vi "Test Virtual Thermometer from CSV.vi"(11 "Test Case In":refnum<class "Test Instrument Manager.lvclass">) -> (0 "error out":errorcluster, 3 "Test Case Out":refnum<class "Test Instrument Manager.lvclass">)   [LabVIEW 2024, in "Test Instrument Manager.lvclass"]
uses:
  Test Instrument Manager.lvclass
  Test Instrument Manager.lvclass/Test Instrument Manager.ctl
  Source/Instrument Manager/Instrument Manager.lvclass
  Source/Interfaces/IRead Temperature/IRead Temperature.lvclass
  Source/Interfaces/IVirtual Instrument/IVirtual Instrument.lvclass
  <vilib>/Astemes/LUnit/Test Case.lvclass
  cceb4bd8-3600-4d38-a702-34d5b4246d90.vi
panel:
  out "Time Stamp":timestamp format="%<%x %.3X>T"
  out "Waveform Chart":dbl(graph)
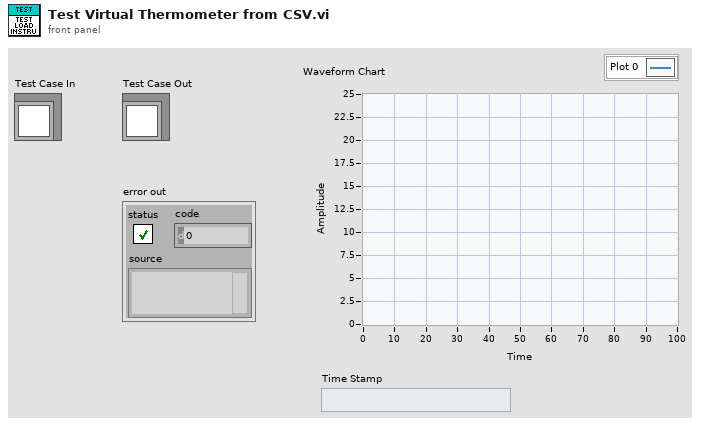
[diagram p1: front panel]
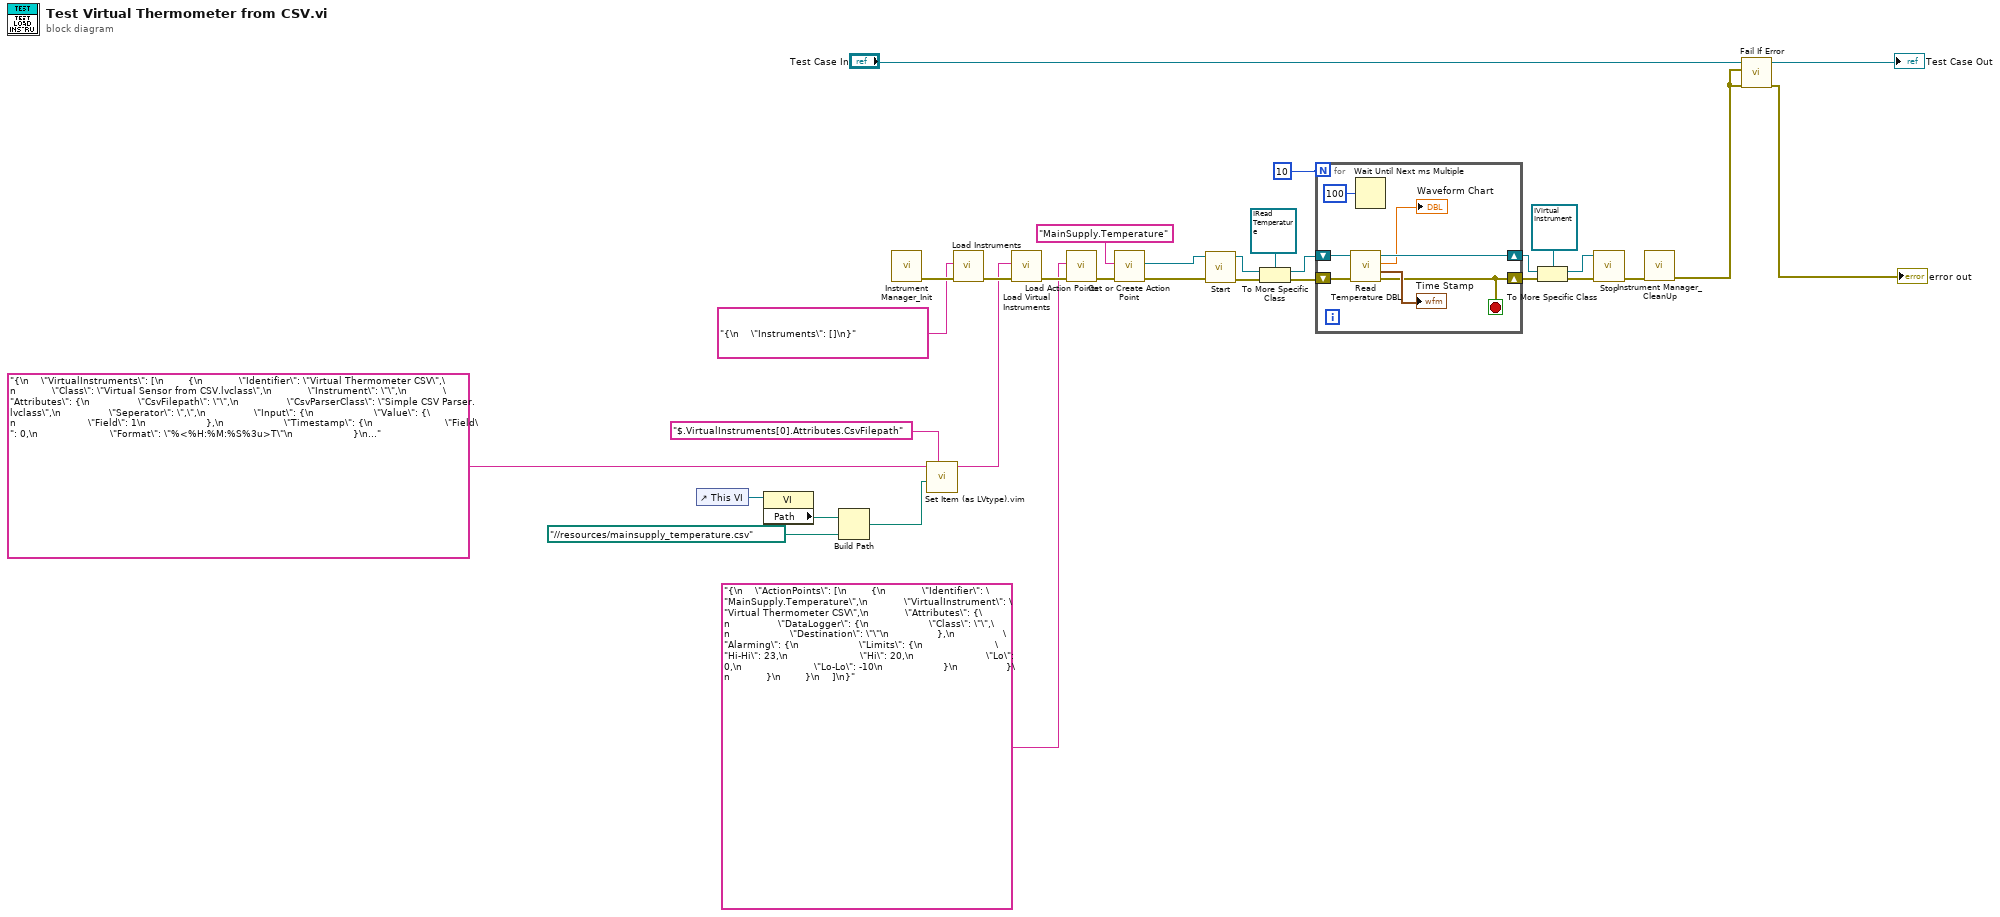
[diagram p0: block diagram]
diagram:
  n1 = control-ref of="This VI"() -> (w5:refnum<vi>)
  n2 = property class="VI"(reference=w5) -> ("Path"=w4:path)  [unwired: 1 in, 2 out]
  n3 = Build Path(base path=w4, name or relative path=path "../../resources/mainsupply_temperature.csv") -> (appended path=w2:path)
  n4 = call "Instrument Manager_Init.vi"() -> ("Error Out"=w30:errorcluster)  [unwired: 10 in, 1 out]
  n5 = call "Set Item (as LVtype).vim"("$Path or Item Name"="$.VirtualInstruments[0].Attributes.CsvFilepath", "Anything"=w2, "JSON"="{\n    \"VirtualInstruments\": [\n        {\n            \"Identifier\": \"Virtual Thermometer CSV\",\n            \"Class\": \"Virtual Sensor from CSV.lvclass\",\n            \"Instrument\": \"\",\n            \"Attributes\": {\n                \"CsvFilepath\": \"\",\n                \"CsvParserClass\": \"Simple CSV Parser.lvclass\",\n                \"Seperator\": \",\",\n                \"Input\": {\n                    \"Value\": {\n                        \"Field\": 1\n                    },\n                    \"Timestamp\": {\n                        \"Field\": 0,\n                        \"Format\": \"%<%H:%M:%S%3u>T\"\n                    }\n                }\n            }\n        }\n    ]\n}") -> ("<JSON>"=w6:string)  [unwired: 5 in, 2 out]
  n6 = call "Load Instruments.vi"("Error In"=w30, "Source"="{\n    \"Instruments\": []\n}") -> ("Error Out"=w29:errorcluster)  [unwired: 9 in]
  n7 = call "Load Virtual Instruments.vi"("Error In"=w29, "Source"=w6) -> ("Error Out"=w26:errorcluster)  [unwired: 9 in]
  n8 = call "Load Action Points.vi"("Error In"=w26, "Source"="{\n    \"ActionPoints\": [\n        {\n            \"Identifier\": \"MainSupply.Temperature\",\n            \"VirtualInstrument\": \"Virtual Thermometer CSV\",\n            \"Attributes\": {\n                \"DataLogger\": {\n                    \"Class\": \"\",\n                    \"Destination\": \"\"\n                },\n                \"Alarming\": {\n                    \"Limits\": {\n                        \"Hi-Hi\": 23,\n                        \"Hi\": 20,\n                        \"Lo\": 0,\n                        \"Lo-Lo\": -10\n                    }\n                }\n            }\n        }\n    ]\n}") -> ("Error Out"=w24:errorcluster)  [unwired: 9 in]
  n9 = call "Get or Create Action Point.vi"("Error In"=w24, "Action Point Identifier"="MainSupply.Temperature") -> ("Error Out"=w21:errorcluster, "IAction Point"=w20:refnum<class "IVirtual Instrument.lvclass">)  [unwired: 8 in]
  n10 = call-dynamic "Start.vi"("error in"=w21, "IRunnable in"=w20) -> ("error out"=w19:errorcluster, "IRunnable out"=w16:refnum<class "IVirtual Instrument.lvclass">)  [unwired: 8 in]
  n11 = To More Specific Class(target class=refnum<class "IRead Temperature.lvclass"> refnum ("IRead Temperature.lvclass"), reference=w16, error in=w19) -> (specific class reference=w14:refnum<class "IRead Temperature.lvclass">, error out=w17:errorcluster)
  n12 = for {
    N: 10 -> [_]
    shift-right: [w33] -> w22
    shift-left: w17 -> [w39]
    shift-right: [w37] -> w12
    shift-left: w14 -> [w38]
    stop <- w33 stop-if-true
    n13 = call-dynamic "Read Temperature DBL.vi"("error in"=w39, "IRead Temperature in"=w38) -> ("error out"=w33:errorcluster, "Time Stamp"=→"Time Stamp":timestamp, "Temperature"=→"Waveform Chart":dbl, "IRead Temperature out"=w37:refnum<class "IRead Temperature.lvclass">)  [unwired: 6 in]
    n14 = Wait Until Next ms Multiple(millisecond multiple=u32 100) -> ()  [unwired: 1 out]
  }
  n15 = To More Specific Class(target class=refnum<class "IVirtual Instrument.lvclass"> refnum ("IVirtual Instrument.lvclass"), reference=w12, error in=w22) -> (specific class reference=w11:refnum<class "IVirtual Instrument.lvclass">, error out=w13:errorcluster)
  n16 = call-dynamic "Stop.vi"("error in"=w13, "IRunnable in"=w11) -> ("error out"=w18:errorcluster)  [unwired: 8 in, 1 out]
  n17 = call "Instrument Manager_CleanUp.vi"("Error In"=w18) -> ("Error Out"=w8:errorcluster)  [unwired: 10 in]
  n18 = call <vilib>:"Fail If Error.vi"("error in (no error)"=w8, "Assert error"=w8, "LUnit Test Case In"="Test Case In") -> ("error out"=→"error out":errorcluster, "LUnit Test Case Out"=→"Test Case Out":refnum<class "Test Instrument Manager.lvclass">)  [unwired: 7 in]
